vi "niRFUtil RFHS Channelizer DesignFilter.vi"(0 "fs":dbl=1.0, 5 "Channel Specification":T1={"fc"=0.0, "fs"=1.0, "passBW"=0.0, "stopBW"=0.0, "Rejection (dB)"=0.0, "Flags"=0, "Reserved"=0} {"Flags" items=["None"=0, "Force Fractional"=1, "Use Multistage"=2, "Use Pretrigger Data "=256, "Frequency Shift Only"=4]; "fs" format="%#_8p"; "fc" format="%#_6p"; "stopBW" format="%#_6p"; "passBW" format="%#_6p"}, 11 "error in (no error)":errorcluster) -> (4 "Filter Taps":dbl[](array[numeric]), 6 "upsample":i32, 8 "downsample":dbl, 15 "error out":errorcluster)   [LabVIEW 2015, in "niRFUtil.lvlib"]
uses:
  niRFUtil.lvlib
  Includes/niRFUtil RFHS Channelizer ChannelSpecificationBase.ctl
  Includes/niRFUtil RFHS Channelizer ChannelFlags.ctl
  <vilib>/Analysis/4window.llb/Kaiser-Bessel Window (DBL).vi
  <vilib>/Analysis/NI_AALPro.lvlib
  <vilib>/Analysis/NI_AALBase.lvlib
panel:
  out "Filter Taps":i32
  out "fpass":dbl
  out "fstop":dbl=0.3
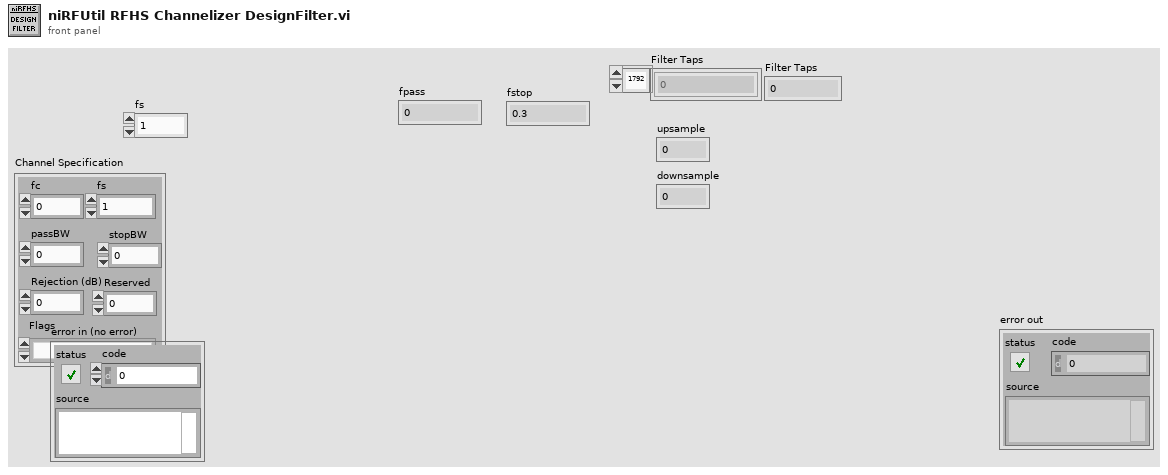
[diagram p1: front panel]
types:
  T1 = typedef "niRFUtil.lvlib/niRFUtil RFHS Channelizer ChannelSpecificationBase.ctl" = cluster{"fc":dbl, "fs":dbl, "passBW":dbl, "stopBW":dbl, "Rejection (dB)":dbl, "Flags":T2, "Reserved":i32}
  T2 = typedef "niRFUtil.lvlib/niRFUtil RFHS Channelizer ChannelFlags.ctl" = u32
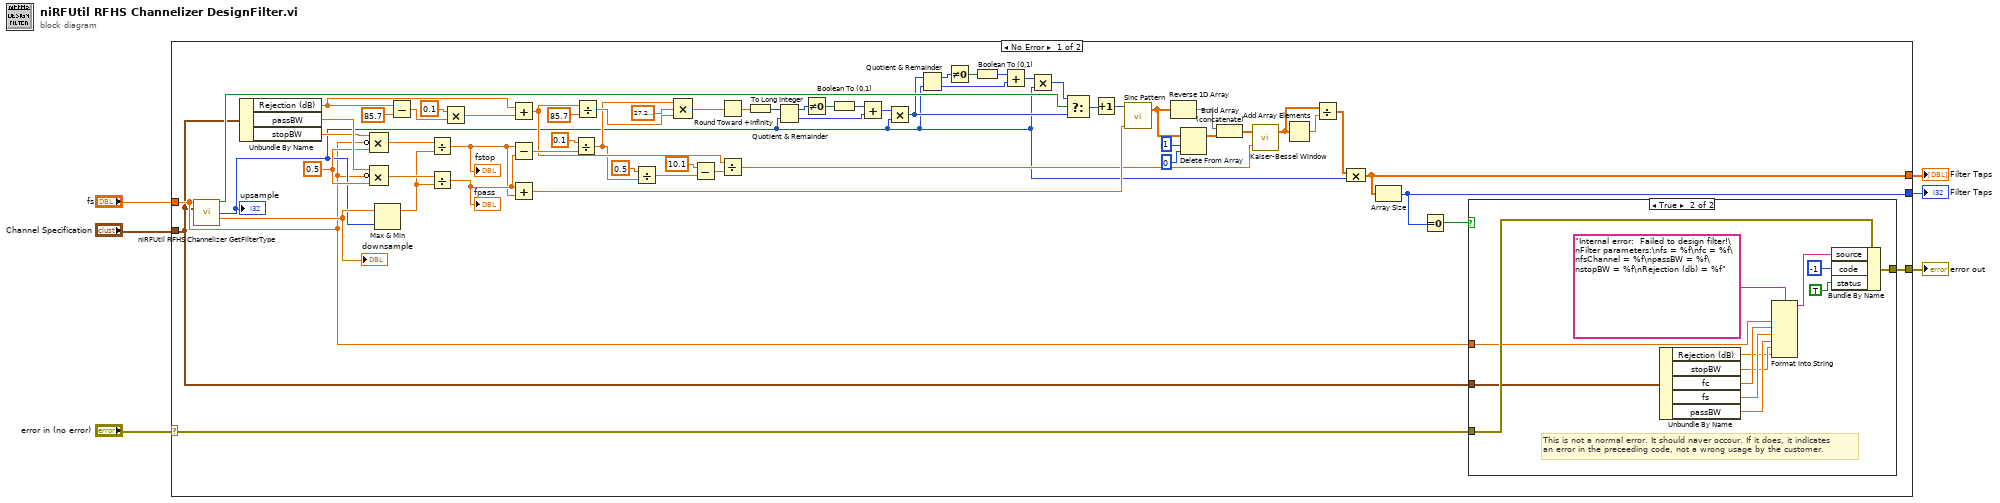
[diagram p0: block diagram]
diagram:
  n1 = case shown="No Error" "error in (no error)" {
    selector: "error in (no error)" -> [w8 w83]
    tunnel: [w12 w83] -> w6
    tunnel: "fs" -> [w11 _]
    tunnel: "Channel Specification" -> [w7 _]
    tunnel: [w10 _] -> w3
    tunnel: [w9 _] -> w2
    frame No Error {
      w29 = 0.5 ("value")
      n2 = call "niRFUtil RFHS Channelizer GetFilterType.vi"("fs"=w11, "Channel Specification"=w7) -> ("Fractional"=w20:bool, "Upsample"=w14:i32, "Downsample"=w15:dbl)  [unwired: 10 in, 1 out]
      "upsample" <- w14
      "downsample" <- w15
      n3 = Unbundle By Name(w7) -> ("Rejection (dB)"=w39:dbl, "passBW"=w44:dbl, "stopBW"=w30:dbl)
      n4 = Compound Arithmetic op=MULTIPLY(w30, invert w11, w29) -> (w28:dbl)
      n5 = Compound Arithmetic op=MULTIPLY(w44, invert w11, w29) -> (w43:dbl)
      n6 = Max & Min(x=w15, y=w14) -> (max(x,y)=w26:dbl)  [unwired: 1 out]
      n7 = Subtract(x=w39, y=85.7) -> (x-y=w53:dbl)
      n8 = Divide(x=w28, y=w26) -> (x/y=w41:dbl)
      "fstop" <- w41
      n9 = Divide(x=w43, y=w26) -> (x/y=w42:dbl)
      "fpass" <- w42
      n10 = Multiply(x=0.1, y=w53) -> (x*y=w51:dbl)
      n11 = Add(x=w39, y=w51) -> (x+y=w50:dbl)
      n12 = Subtract(x=w41, y=w42) -> (x-y=w62:dbl)
      n13 = Add(x=w42, y=w41) -> (x+y=w60:dbl)
      n14 = Divide(x=0.1 ("y"), y=w62) -> (x/y=w46:dbl)
      n15 = Divide(x=w50, y=85.7) -> (x/y=w56:dbl)
      n16 = Divide(x=0.5, y=w46) -> (x/y=w48:dbl)
      n17 = Compound Arithmetic op=MULTIPLY(w46, sgl 27.2 ("y"), w56) -> (w40:dbl)
      n18 = Subtract(x=10.1, y=w48) -> (x-y=w45:dbl)
      n19 = Round Toward +Infinity(x=w40) -> (ceil(x): smallest int >= x=w31:dbl)
      n20 = Divide(x=w50, y=w45) -> (x/y=w55:dbl)
      n21 = To Long Integer(number=w31) -> (32bit integer=w17:i32)
      n22 = Quotient & Remainder(x=w17, y=w14) -> (x-y*floor(x/y)=w36:i32, floor(x/y)=w33:i32)
      n23 = Not Equal To 0?(x=w36) -> (x != 0?=w35:bool)
      n24 = Boolean To (0,1)(Boolean=w35) -> (0, 1=w34:i16)
      n25 = Add(x=w34, y=w33) -> (x+y=w32:i32)
      n26 = Multiply(x=w32, y=w14) -> (x*y=w18:i32)
      n27 = Quotient & Remainder(x=w18, y=w14) -> (x-y*floor(x/y)=w21:i32, floor(x/y)=w24:i32)
      n28 = Not Equal To 0?(x=w21) -> (x != 0?=w22:bool)
      n29 = Boolean To (0,1)(Boolean=w22) -> (0, 1=w23:i16)
      n30 = Add(x=w23, y=w24) -> (x+y=w25:i32)
      n31 = Multiply(x=w25, y=w14) -> (x*y=w19:i32)
      n32 = Select(t=w19, s=w20, f=w18) -> (s? t:f=w16:i32)
      n33 = Increment(x=w16) -> (x+1=w27:i32)
      n34 = call <vilib>:"Sinc Pattern.vi"("delta t"=w60, "samples"=w27) -> ("Sinc Pattern"=w61:dbl[])  [unwired: 2 in, 1 out]
      n35 = Reverse 1D Array(array=w61) -> (reversed array=w66:dbl[])
      n36 = Delete From Array(array=w61, length=1, index=0) -> (array with subset deleted=w65:dbl[])  [unwired: 1 out]
      n37 = Build Array (concatenate)(w66, w65) -> (w58:dbl[])
      n38 = call-poly <vilib>:"Kaiser-Bessel Window.vi"("beta"=w55, "X"=w58) -> ("Windowed X"=w38:dbl[])  [unwired: 1 out]
      n39 = Add Array Elements(numeric array=w38) -> (sum=w59:dbl)
      n40 = Divide(x=w38, y=w59) -> (x/y=w37:dbl[])
      n41 = Compound Arithmetic op=MULTIPLY(w37, w14) -> (w10:dbl[])
      n42 = Array Size(array=w10) -> (size(s)=w9:i32)
      n43 = Equal To 0?(x=w9) -> (x = 0?=w13:bool)
      n44 = case shown="True" w13 {
        tunnel: w8 -> [w69 w82]
        tunnel: [w69 w81] -> w12
        tunnel: w11 -> [_ w76]
        tunnel: w7 -> [_ w77]
        frame False {
        }
        frame True {
          # "This is not a normal error. It should naver occour. If it does, it indicates \nan error in the preceeding code, not a wrong usage by the customer."
          n45 = Unbundle By Name(w77) -> ("Rejection (dB)"=w70:dbl, "stopBW"=w72:dbl, "fc"=w75:dbl, "fs"=w74:dbl, "passBW"=w73:dbl)
          n46 = Format Into String(format string="Internal error:  Failed to design filter!\nFilter parameters:\nfs = %f\nfc = %f\nfsChannel = %f\npassBW = %f\nstopBW = %f\nRejection (db) = %f", w76, w75, w74, w73, w72, w70) -> (resulting string=w78:string)  [unwired: 2 in, 1 out]
          n47 = Bundle By Name(cluster=w82, "source"=w78, "code"=-1, "status"=TRUE) -> (w81:errorcluster)
        }
      }
    }
    frame Error {
    }
  }
  "error out" <- w6
  "Filter Taps" <- w3
  "Filter Taps" <- w2
